vi "Car_wash.vi"() -> ()   [LabVIEW 2020]
uses:
  Wash options.ctl
panel:
  out "Cars in queue":u32
  in  "stop":bool
  out "Position":i32(slide) scale=0.0..5.0
  out "Number of cars in queue":u8(slide) scale=0.0..20.0
  out "Name of the Owner.":string
  in  "Start":bool
  in  "Name of the Owner":string
  out "Status":T1
  in  "Wash options":T2
  # "Start"
  # "Station 1\nUnderbody wash\nPre-soak"
  # "Station 2 \nHigh-pressure wash\nLow-pressure wash\nRinse"
  # "Station 3\nWaxing\nPolishing"
  # "Station 4\nAir Dry"
  # "End"
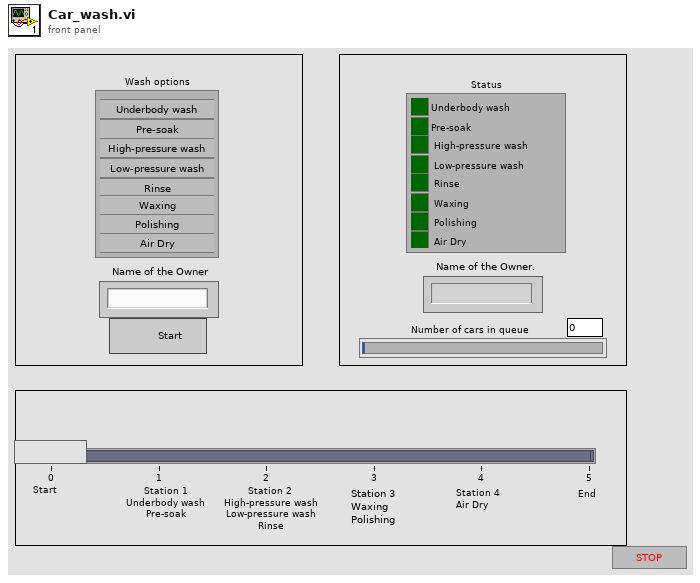
[diagram p1: front panel]
types:
  T1 = cluster{"Underbody wash":bool, "Pre-soak":bool, " High-pressure wash":bool, " Low-pressure wash":bool, " Rinse":bool, " Waxing":bool, " Polishing":bool, " Air Dry":bool}
  T2 = cluster{"Underbody wash":bool, "Pre-soak":bool, "High-pressure wash":bool, "Low-pressure wash":bool, "Rinse":bool, "Waxing":bool, "Polishing":bool, "Air Dry":bool}
  T3 = typedef "Wash options.ctl" = enum16{"Start", "1", "1.5", "2", "2.3", "2.7", "3", "3.5", "4", "End", "Init"}
  T4 = cluster{"element":cluster{"Underbody wash":bool, "Pre-soak":bool, "High-pressure wash":bool, "Low-pressure wash":bool, "Rinse":bool, "Waxing":bool, "Polishing":bool, "Air Dry":bool}, string, T3}
  T5 = cluster{"Wash options":cluster{"Underbody wash":bool, "Pre-soak":bool, "High-pressure wash":bool, "Low-pressure wash":bool, "Rinse":bool, "Waxing":bool, "Polishing":bool, "Air Dry":bool}, "Name of the Owner":string, T3}
  T6 = cluster{"Underbody wash":bool, "Underbody wash":bool, bool, bool, bool, bool, bool, bool}
  T7 = cluster{"Underbody wash":bool, "Pre-soak":bool, bool, bool, bool, bool, bool, bool}
  T8 = cluster{bool, bool, bool, bool, bool, bool, bool, bool}
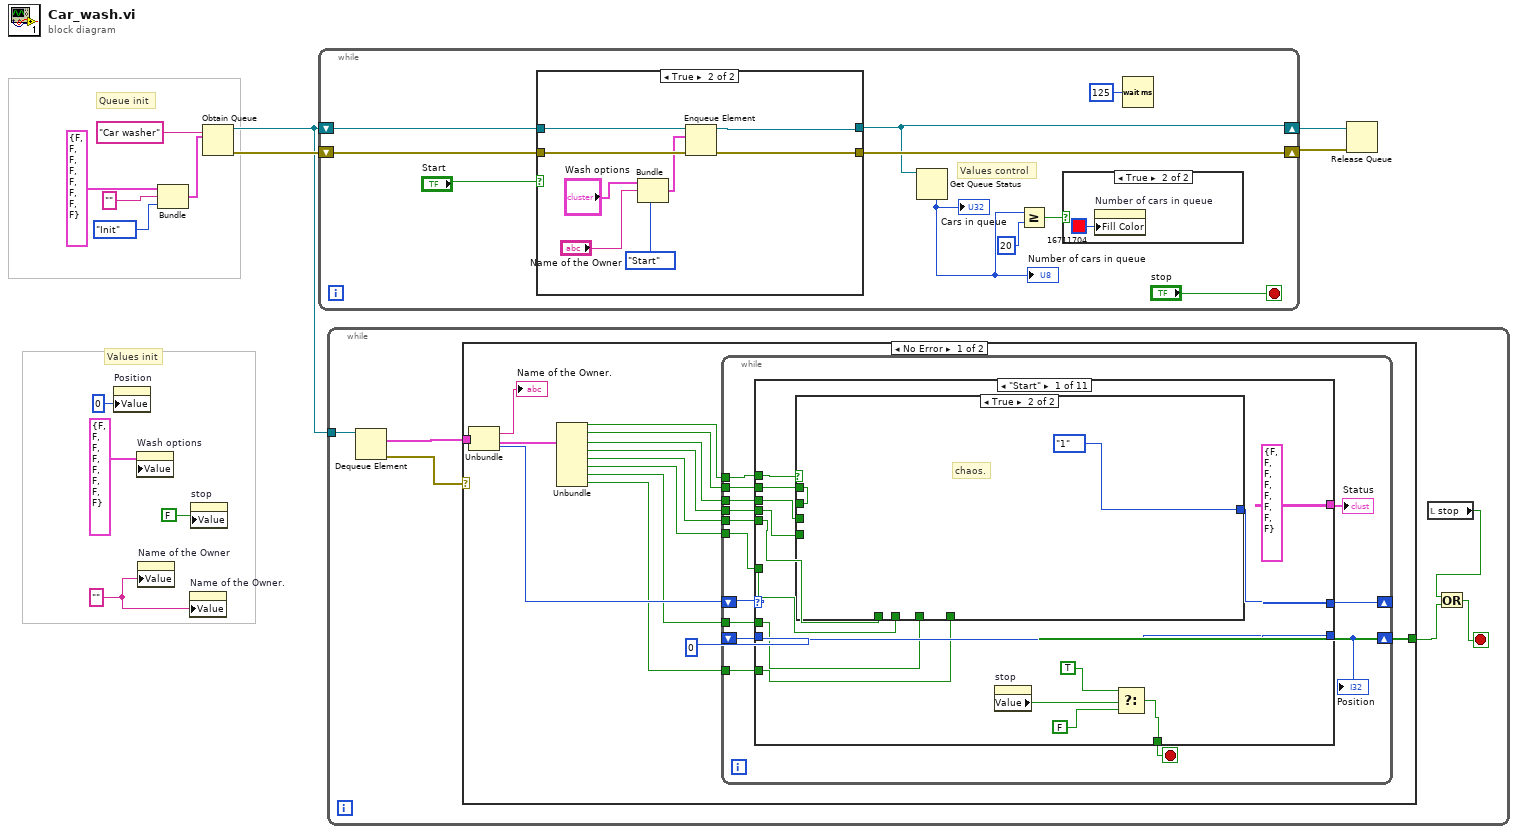
[diagram p0: block diagram]
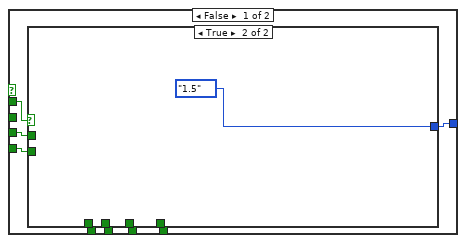
[diagram p2: hidden frame]
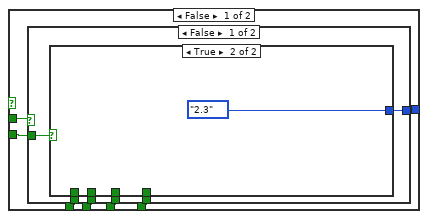
[diagram p3: hidden frame]
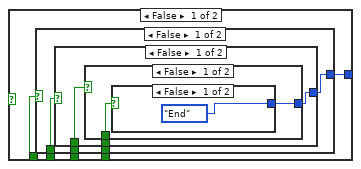
[diagram p4: hidden frame]
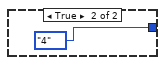
[diagram p5: hidden frame]
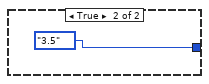
[diagram p6: hidden frame]
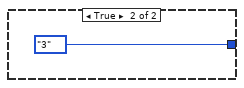
[diagram p7: hidden frame]
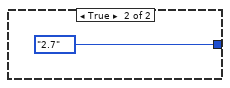
[diagram p8: hidden frame]
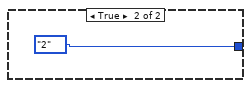
[diagram p9: hidden frame]
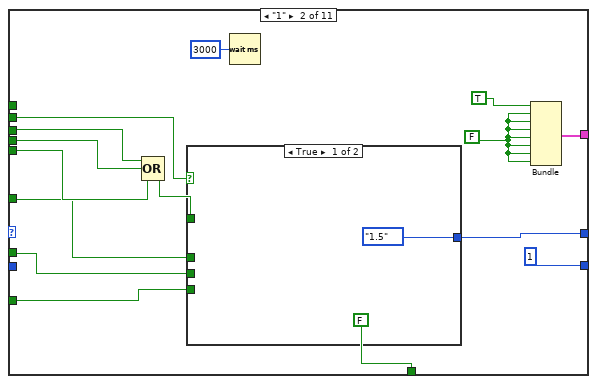
[diagram p10: hidden frame]
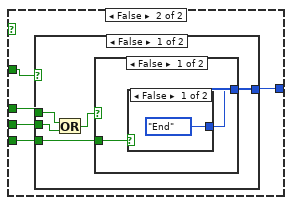
[diagram p11: hidden frame]
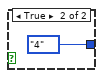
[diagram p12: hidden frame]
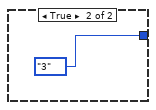
[diagram p13: hidden frame]
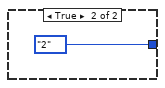
[diagram p14: hidden frame]
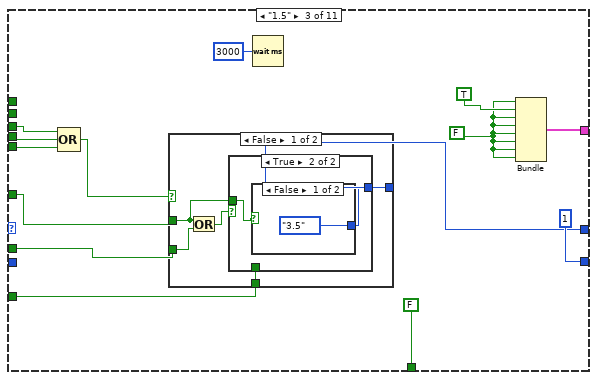
[diagram p15: hidden frame]
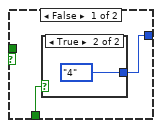
[diagram p16: hidden frame]
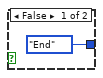
[diagram p17: hidden frame]
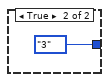
[diagram p18: hidden frame]
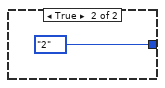
[diagram p19: hidden frame]
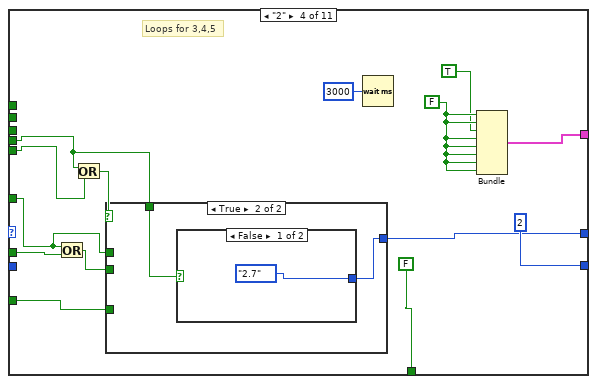
[diagram p20: hidden frame]
diagram:
  w2 = "" ("Name of the Owner")
  # "Values init"
  # "Queue init"
  n1 = property on="Position" class="Slide (strict)"("Value"=0 ("Position")) -> ()  [unwired: 2 in, 2 out]
  n2 = property on="Wash options" class="Clust (strict)"("Value"=T2 {"Underbody wash"=FALSE, "Pre-soak"=FALSE, "High-pressure wash"=FALSE, "Low-pressure wash"=FALSE, "Rinse"=FALSE, "Waxing"=FALSE, "Polishing"=FALSE, "Air Dry"=FALSE} ("Wash options")) -> ()  [unwired: 2 in, 2 out]
  n3 = property on="Name of the Owner" class="Str"("Value"=w2) -> ()  [unwired: 2 in, 2 out]
  n4 = Bundle("element"=T2 {"Underbody wash"=FALSE, "Pre-soak"=FALSE, "High-pressure wash"=FALSE, "Low-pressure wash"=FALSE, "Rinse"=FALSE, "Waxing"=FALSE, "Polishing"=FALSE, "Air Dry"=FALSE}, "", Wash_options."Init") -> (w6:T4)  [unwired: 1 in]
  n5 = property on="Name of the Owner." class="Str"("Value"=w2) -> ()  [unwired: 2 in, 2 out]
  n6 = property on="stop" class="Bool (strict)"("Value"=FALSE ("stop")) -> ()  [unwired: 2 in, 2 out]
  n7 = Obtain Queue(name (unnamed)="Car washer", element data type=w6) -> (queue out=w9:refnum<queue>, error out=w10:errorcluster)  [unwired: 3 in, 1 out]
  n8 = while {
    shift-right: [w22] -> w11
    shift-left: w10 -> [w21]
    shift-right: [w18] -> w12
    shift-left: w9 -> [w14]
    stop <- "stop" stop-if-true
    # "Values control"
    n9 = case shown="True" "Start" {
      tunnel: [w27 w28] -> w18
      tunnel: w14 -> [w27 w35]
      tunnel: [w26 w34] -> w22
      tunnel: w21 -> [w26 w33]
      frame False {
      }
      frame True {
        n10 = Bundle("Wash options"="Wash options", "Name of the Owner"="Name of the Owner", Wash_options."Start") -> (w31:T5)  [unwired: 1 in]
        n11 = Enqueue Element(queue=w35, element=w31, error in (no error)=w33) -> (queue out=w28:refnum<queue>, error out=w34:errorcluster)  [unwired: 1 in, 1 out]
      }
    }
    n12 = Get Queue Status(queue=w18) -> (# elements in queue=w17:i32)  [unwired: 2 in, 7 out]
    "Cars in queue" <- w17
    "Number of cars in queue" <- w17
    n13 = Greater Or Equal?(x=w17, y=20) -> (x >= y?=w15:bool)
    n14 = case shown="True" w15 {
      frame False {
        n15 = property on="Number of cars in queue" class="Slide (strict)"("Fill Color"=u32 23039) -> ()  [unwired: 2 in, 2 out]
      }
      frame True {
        n16 = property on="Number of cars in queue" class="Slide (strict)"("Fill Color"=u32 16711704) -> ()  [unwired: 2 in, 2 out]
      }
    }
    n17 = Wait (ms)(milliseconds to wait=u32 125) -> ()  [unwired: 1 out]
  }
  n18 = while {
    tunnel: w9 -> [w39]
    stop <- w37 stop-if-true
    n19 = Dequeue Element(queue=w39) -> (element=w40:T4, error out=w41:errorcluster)  [unwired: 2 in, 2 out]
    n20 = case shown="No Error" w41 {
      selector: w41 -> [_ w306]
      tunnel: w40 -> [w54 _]
      tunnel: [_ TRUE] -> w38
      frame No Error {
        n21 = Unbundle(w54) -> ("element"=w53:T2, →"Name of the Owner.":string, w49:T3)
        n22 = Unbundle(w53) -> ("Underbody wash"=w52:bool, "Pre-soak"=w51:bool, "High-pressure wash"=w48:bool, "Low-pressure wash"=w47:bool, "Rinse"=w46:bool, "Waxing"=w45:bool, "Polishing"=w44:bool, "Air Dry"=w42:bool)
        n23 = while {
          tunnel: w52 -> [w67]
          tunnel: w51 -> [w66]
          shift-right: [w64] -> _
          shift-left: 0 -> [w65]
          shift-right: [w62] -> _
          shift-left: w49 -> [w63]
          tunnel: w48 -> [w60]
          tunnel: w47 -> [w59]
          tunnel: w46 -> [w58]
          tunnel: w45 -> [w57]
          tunnel: w44 -> [w56]
          tunnel: w42 -> [w55]
          stop <- w61 stop-if-true
          n24 = case shown="\"Start\"" w63 {
            selector: w63 -> [_ _ _ _ _ _ _ _ _ _ w305]
            tunnel: [T6 {"Underbody wash"=FALSE, "Underbody wash"=FALSE, FALSE, FALSE, FALSE, FALSE, FALSE, FALSE} w142 w173 w198 w224 w249 w268 w283 w286 T7 {"Underbody wash"=FALSE, "Pre-soak"=FALSE, FALSE, FALSE, FALSE, FALSE, FALSE, FALSE} T7 {"Underbody wash"=FALSE, "Pre-soak"=FALSE, FALSE, FALSE, FALSE, FALSE, FALSE, FALSE}] -> w68
            tunnel: w67 -> [w80 _ _ _ _ _ _ _ _ _ _]
            tunnel: w66 -> [w73 w129 _ _ _ _ _ _ _ _ _]
            tunnel: w65 -> [w82 _ _ _ _ _ _ _ _ _ _]
            tunnel: [w82 1 1 2 2 2 3 3 4 5 0] -> w64
            tunnel: [w81 w135 w170 w196 w222 w245 w265 w278 Wash_options."End" Wash_options."Init" w305] -> w62
            tunnel: [w70 FALSE FALSE FALSE FALSE FALSE FALSE FALSE FALSE w295 TRUE] -> w61
            tunnel: w60 -> [w79 w139 w169 _ _ _ _ _ _ _ _]
            tunnel: w59 -> [w78 w138 w168 w192 _ _ _ _ _ _ _]
            tunnel: w58 -> [w74 w137 w167 w193 w223 _ _ _ _ _ _]
            tunnel: w57 -> [w77 w134 w165 w188 w221 w243 _ _ _ _ _]
            tunnel: w56 -> [w76 w133 w164 w197 w220 w247 w262 _ _ _ _]
            tunnel: w55 -> [w75 w132 w163 w195 w219 w244 w266 w279 _ _ _]
            frame "Start" {
              n25 = case shown="True" w80 {
                tunnel: [w89 Wash_options."1"] -> w81
                tunnel: w73 -> [_ _]
                tunnel: w79 -> [w91 _]
                tunnel: w78 -> [w90 _]
                tunnel: w74 -> [w88 _]
                tunnel: w77 -> [w87 _]
                tunnel: w76 -> [w86 _]
                tunnel: w75 -> [w85 _]
                tunnel: w73 -> [w84 _]
                frame False {
                  n26 = case shown="True" w84 {
                    tunnel: w91 -> [w98 _]
                    tunnel: w90 -> [w97 _]
                    tunnel: [w96 Wash_options."1.5"] -> w89
                    tunnel: w88 -> [w95 _]
                    tunnel: w87 -> [w94 _]
                    tunnel: w86 -> [w93 _]
                    tunnel: w85 -> [w92 _]
                    frame False {
                      n27 = case shown="False" w98 {
                        tunnel: w97 -> [w104 _]
                        tunnel: [w103 Wash_options."2"] -> w96
                        tunnel: w95 -> [w102 _]
                        tunnel: w94 -> [w101 _]
                        tunnel: w93 -> [w100 _]
                        tunnel: w92 -> [w99 _]
                        frame False {
                          n28 = case shown="True" w104 {
                            tunnel: [w108 Wash_options."2.3"] -> w103
                            tunnel: w102 -> [w109 _]
                            tunnel: w101 -> [w107 _]
                            tunnel: w100 -> [w106 _]
                            tunnel: w99 -> [w105 _]
                            frame False {
                              n29 = case shown="False" w109 {
                                tunnel: [w112 Wash_options."2.7"] -> w108
                                tunnel: w107 -> [w113 _]
                                tunnel: w106 -> [w111 _]
                                tunnel: w105 -> [w110 _]
                                frame False {
                                n30 = case shown="False" w113 {
                                tunnel: [w115 Wash_options."3"] -> w112
                                tunnel: w111 -> [w116 _]
                                tunnel: w110 -> [w114 _]
                                frame False {
                                n31 = case shown="False" w116 {
                                tunnel: [w117 Wash_options."3.5"] -> w115
                                tunnel: w114 -> [w118 _]
                                frame False {
                                n32 = case shown="False" w118 {
                                tunnel: [Wash_options."End" Wash_options."4"] -> w117
                                frame False {
                                }
                                frame True {
                                }
                                }
                                }
                                frame True {
                                }
                                }
                                }
                                frame True {
                                }
                                }
                                }
                                frame True {
                                }
                              }
                            }
                            frame True {
                            }
                          }
                        }
                        frame True {
                        }
                      }
                    }
                    frame True {
                    }
                  }
                }
                frame True {
                  # "chaos."
                }
              }
              n33 = property on="stop" class="Bool (strict)"() -> ("Value"=w69:bool)  [unwired: 2 in, 2 out]
              n34 = Select(t=TRUE, s=w69, f=FALSE) -> (s? t:f=w70:bool)
            }
            frame "1" {
              w131 = FALSE
              n35 = Compound Arithmetic op=OR(w139, w138, w137) -> (w136:bool)
              n36 = case shown="True" w129 {
                tunnel: w136 -> [_ w148]
                tunnel: [Wash_options."1.5" w147] -> w135
                tunnel: w134 -> [_ w146]
                tunnel: w133 -> [_ w145]
                tunnel: w132 -> [_ w144]
                frame True {
                }
                frame False {
                  n37 = case shown="False" w148 {
                    tunnel: [w150 Wash_options."2"] -> w147
                    tunnel: w146 -> [w152 _]
                    tunnel: w145 -> [w151 _]
                    tunnel: w144 -> [w149 _]
                    frame False {
                      n38 = Or(x=w152, y=w151) -> (x .or. y?=w153:bool)
                      n39 = case shown="False" w153 {
                        tunnel: [w154 Wash_options."3"] -> w150
                        tunnel: w149 -> [w155 _]
                        frame False {
                          n40 = case shown="False" w155 {
                            tunnel: [Wash_options."End" Wash_options."4"] -> w154
                            frame False {
                            }
                            frame True {
                            }
                          }
                        }
                        frame True {
                        }
                      }
                    }
                    frame True {
                    }
                  }
                }
              }
              n41 = Wait (ms)(milliseconds to wait=u32 3000) -> ()  [unwired: 1 out]
              n42 = Bundle(TRUE, w131, w131, w131, w131, w131, w131, w131) -> (w142:T8)  [unwired: 1 in]
            }
            frame "1.5" {
              w160 = FALSE
              n43 = Compound Arithmetic op=OR(w169, w168, w167) -> (w166:bool)
              n44 = case shown="False" w166 {
                tunnel: [w177 Wash_options."2"] -> w170
                tunnel: w165 -> [w174 _]
                tunnel: w164 -> [w176 _]
                tunnel: w163 -> [w175 _]
                frame False {
                  n45 = Or(x=w174, y=w176) -> (x .or. y?=w178:bool)
                  n46 = case shown="True" w178 {
                    tunnel: [w180 w183] -> w177
                    tunnel: w175 -> [w179 _]
                    tunnel: w174 -> [_ w184]
                    frame False {
                      n47 = case shown="True" w179 {
                        tunnel: [Wash_options."End" Wash_options."4"] -> w180
                        frame False {
                        }
                        frame True {
                        }
                      }
                    }
                    frame True {
                      n48 = case shown="False" w184 {
                        tunnel: [Wash_options."3.5" Wash_options."3"] -> w183
                        frame False {
                        }
                        frame True {
                        }
                      }
                    }
                  }
                }
                frame True {
                }
              }
              n49 = Wait (ms)(milliseconds to wait=u32 3000) -> ()  [unwired: 1 out]
              n50 = Bundle(w160, TRUE, w160, w160, w160, w160, w160, w160) -> (w173:T8)  [unwired: 1 in]
            }
            frame "2" {
              w191 = FALSE
              # "Loops for 3,4,5"
              n51 = Or(x=w188, y=w197) -> (x .or. y?=w189:bool)
              n52 = Or(x=w192, y=w193) -> (x .or. y?=w194:bool)
              n53 = case shown="True" w194 {
                tunnel: w189 -> [w205 _]
                tunnel: [w204 w214] -> w196
                tunnel: w195 -> [w203 _]
                tunnel: w192 -> [_ w215]
                tunnel: w188 -> [w202 _]
                frame False {
                  n54 = case shown="False" w205 {
                    tunnel: [w206 w210] -> w204
                    tunnel: w203 -> [w207 _]
                    tunnel: w202 -> [_ w211]
                    frame False {
                      n55 = case shown="True" w207 {
                        tunnel: [Wash_options."End" Wash_options."4"] -> w206
                        frame False {
                        }
                        frame True {
                        }
                      }
                    }
                    frame True {
                      n56 = case shown="True" w211 {
                        tunnel: [Wash_options."3.5" Wash_options."3"] -> w210
                        frame False {
                        }
                        frame True {
                        }
                      }
                    }
                  }
                }
                frame True {
                  n57 = case shown="False" w215 {
                    tunnel: [Wash_options."2.7" Wash_options."2.3"] -> w214
                    frame False {
                    }
                    frame True {
                    }
                  }
                }
              }
              n58 = Wait (ms)(milliseconds to wait=u32 3000) -> ()  [unwired: 1 out]
              n59 = Bundle(w191, w191, TRUE, w191, w191, w191, w191, w191) -> (w198:T8)  [unwired: 1 in]
            }
            frame "2.3" {
              w226 = FALSE
              n60 = case shown="False" w223 {
                tunnel: [w231 Wash_options."2.7"] -> w222
                tunnel: w221 -> [w229 _]
                tunnel: w220 -> [w233 _]
                tunnel: w219 -> [w230 _]
                frame False {
                  n61 = Or(x=w229, y=w233) -> (x .or. y?=w232:bool)
                  n62 = case shown="False" w232 {
                    tunnel: [w234 w238] -> w231
                    tunnel: w230 -> [w235 _]
                    tunnel: w229 -> [_ w239]
                    frame False {
                      n63 = case shown="True" w235 {
                        tunnel: [Wash_options."End" Wash_options."4"] -> w234
                        frame False {
                        }
                        frame True {
                        }
                      }
                    }
                    frame True {
                      n64 = case shown="False" w239 {
                        tunnel: [Wash_options."3.5" Wash_options."3"] -> w238
                        frame False {
                        }
                        frame True {
                        }
                      }
                    }
                  }
                }
                frame True {
                }
              }
              n65 = Wait (ms)(milliseconds to wait=u32 3000) -> ()  [unwired: 1 out]
              n66 = Bundle(w226, w226, w226, TRUE, w226, w226, w226, w226) -> (w224:T8)  [unwired: 1 in]
            }
            frame "2.7" {
              w251 = FALSE
              n67 = Or(x=w243, y=w247) -> (x .or. y?=w246:bool)
              n68 = case shown="False" w246 {
                tunnel: [w254 w258] -> w245
                tunnel: w244 -> [w255 _]
                tunnel: w243 -> [_ w259]
                frame False {
                  n69 = case shown="False" w255 {
                    tunnel: [Wash_options."End" Wash_options."4"] -> w254
                    frame False {
                    }
                    frame True {
                    }
                  }
                }
                frame True {
                  n70 = case shown="False" w259 {
                    tunnel: [Wash_options."3.5" Wash_options."3"] -> w258
                    frame False {
                    }
                    frame True {
                    }
                  }
                }
              }
              n71 = Wait (ms)(milliseconds to wait=u32 3000) -> ()  [unwired: 1 out]
              n72 = Bundle(w251, w251, w251, w251, TRUE, w251, w251, w251) -> (w249:T8)  [unwired: 1 in]
            }
            frame "3" {
              w263 = FALSE
              # "Loops for 6,7"
              n73 = Wait (ms)(milliseconds to wait=u32 3000) -> ()  [unwired: 1 out]
              n74 = case shown="True" w262 {
                tunnel: w266 -> [w272 _]
                tunnel: [w271 Wash_options."3.5"] -> w265
                frame False {
                  n75 = case shown="True" w272 {
                    tunnel: [Wash_options."End" Wash_options."4"] -> w271
                    frame False {
                    }
                    frame True {
                    }
                  }
                }
                frame True {
                }
              }
              n76 = Bundle(w263, w263, w263, w263, w263, TRUE, w263, w263) -> (w268:T8)  [unwired: 1 in]
            }
            frame "3.5" {
              w282 = FALSE
              n77 = case shown="False" w279 {
                tunnel: [Wash_options."End" Wash_options."4"] -> w278
                frame False {
                }
                frame True {
                }
              }
              n78 = Wait (ms)(milliseconds to wait=u32 3000) -> ()  [unwired: 1 out]
              n79 = Bundle(w282, w282, w282, w282, w282, w282, TRUE, w282) -> (w283:T8)  [unwired: 1 in]
            }
            frame "4" {
              w288 = FALSE
              # "Loop for last value"
              n80 = Wait (ms)(milliseconds to wait=u32 3000) -> ()  [unwired: 1 out]
              n81 = Bundle(w288, w288, w288, w288, w288, w288, w288, TRUE) -> (w286:T8)  [unwired: 1 in]
            }
            frame "End" {
              # "Ending values, closing state machine"
              n82 = Wait (ms)(milliseconds to wait=u32 3000) -> ()  [unwired: 1 out]
              n83 = property on="stop" class="Bool (strict)"() -> ("Value"=w296:bool)  [unwired: 2 in, 2 out]
              n84 = Select(t=TRUE, s=w296, f=FALSE) -> (s? t:f=w295:bool)
            }
            frame "Init", Default {
              # "The loop is off"
              # "Beginning values"
              # "Doing nothing"
              n85 = Wait (ms)(milliseconds to wait=u32 125) -> ()  [unwired: 1 out]
            }
          }
          "Status" <- w68
          "Position" <- w64
        }
      }
      frame Error {
        # "In case of any error"
        n86 = call <vilib>:"Simple Error Handler.vi"("error in (no error)"=w306) -> ()  [unwired: 4 in, 5 out]
      }
    }
    n87 = local read "stop"() -> (w36:bool)
    n88 = Or(x=w36, y=w38) -> (x .or. y?=w37:bool)
  }
  n89 = Release Queue(queue=w12, error in (no error)=w11) -> ()  [unwired: 1 in, 3 out]
